vi "Measurement UI.vi"() -> ()   [LabVIEW 2021, in "Sweep_Channel Ganging.lvlib"]
uses:
  Sweep_Channel Ganging.lvlib
panel:
  in  "MeasGraphs":enum32{"I-V Sweep", "Hidden Controls"}(tab)
  out "LoadGraph":T1(graph)
  out "SourceGraph":T2(graph)
  in  "Load measure trigger":string
  in  "Load source trigger":string
  out "Ganged source currents":dbl[](array[numeric])
  out "Ganged source voltages":dbl[](array[numeric])
  out "Ganged load currents":dbl[](array[numeric])
  out "Ganged load voltages":dbl[](array[numeric])
  in  "Load slave resource names":string[](array[string])
  in  "Load master resource name":string
  in  "Source slave resource names":string[](array[string])
  in  "Source master resource name":string
  out "Load sweep points":i32
  out "Source sweep points":i32
  in  "MeasConfigurations":enum32{"Source Config", "Load Config"}(tab)
  in  "Source ON/OFF":bool=TRUE
  in  "Source source delay":dbl=0.005 caption="SOURCE DELAY" format="%.3ps"
  in  "PPSSlaveResourceNames":refnum<k15>[](array[refnum]) caption="SLAVE RESOURCE NAMES"
  in  "PPSMasterResourceName":refnum<k15> caption="MASTER RESOURCE NAME"
  in  "Source stop level":dbl=20.0 caption="STOP LEVEL" format="%#_6pV"
  in  "Source transient response":i32(ring)=1038 caption="TRANSIENT RESPONSE" items=["Slow"=1041, "Normal"=1038, "Fast"=1039]
  in  "Source sense":i32(ring)=1009 caption="SENSE" items=["Local"=1008, "Remote"=1009]
  in  "Source voltage/current level range":dbl=20.0 caption="VOLTAGE LEVEL RANGE" format="%#_6pV"
  in  "Source start level":dbl=6.0 caption="START LEVEL" format="%#_6pV"
  in  "Source current/voltage limit high":dbl=25.0 caption="CURRENT LIMIT/LIMIT HIGH" format="%#_6pA"
  in  "Source current/voltage limit range":dbl=25.0 caption="CURRENT LIMIT RANGE" format="%#_6pA"
  in  "Source limit symmetry":enum32{"Symmetric", "Asymmetric"}(ring)=enum."Asymmetric" caption="LIMIT SYMMETRY"
  in  "Source current/voltage limit low":dbl=-0.6 caption="CURRENT LIMIT LOW" format="%#_6pA"
  in  "Source system configuration":enum32{"Series", "Parallel"}(ring)=enum."Parallel" caption="SYSTEM CONFIG"
  in  "Source compliance":string="Compliance"
  in  "Source sourceadapt":string="SourceAdapt"
  in  "Source sweep points/points per decade":i32=4 caption="PTS/PTS PER DECADE"
  in  "Source output function":i32(ring)=1006 caption="OUTPUT FUNCTION" items=["DC Voltage"=1006, "DC Current"=1007]
  in  "Source timing":string="Timings"
  in  "Source aperture time":dbl=0.01666 caption="APERTURE TIME" format="%.3ps"
  in  "Source sweep scale":string(combo)="Linear" caption="SCALE"
  in  "Load Source Trigger":tag caption="SOURCE TRIGGER"
  in  "Load aperture time":dbl=0.01666 caption="APERTURE TIME" format="%.3ps"
  in  "Load Measure Trigger":tag caption="MEASURE TRIGGER"
  in  "Load trigger config":string="Trigger"
  in  "Load timing":string="Timings"
  in  "Load output function":i32(ring)=1007 caption="OUTPUT FUNCTION" items=["DC Voltage"=1006, "DC Current"=1007]
  in  "Load sweep points/points per decade":i32=10 caption="PTS/PTS PER DECADE"
  in  "Load stop level":dbl=50.0 caption="STOP LEVEL" format="%#_6pA"
  in  "Load sourceadapt":string="SourceAdapt"
  in  "Load compliance":string="Compliance"
  in  "Load system configuration":enum32{"Series", "Parallel"}(ring)=enum."Parallel" caption="SYSTEM CONFIG"
  in  "Load current/voltage limit low":dbl caption="VOLTAGE  LIMIT LOW" format="%#_6pV"
  in  "Load limit symmetry":enum32{"Symmetric", "Asymmetric"}(ring) caption="LIMIT SYMMETRY"
  in  "Load current/voltage limit range":dbl=6.0 caption="VOLTAGE LIMIT RANGE" format="%#_6pV"
  in  "Load current/voltage limit high":dbl=inf caption="VOLTAGE LIMIT/LIMIT HIGH" format="%#_6p"
  in  "Load start level":dbl=2.0 caption="START LEVEL" format="%#_6pA"
  in  "Load voltage/current level range":dbl=80.0 caption="CURRENT LEVEL RANGE" format="%#_6pA"
  in  "Load sense":i32(ring)=1009 caption="SENSE" items=["Local"=1008, "Remote"=1009]
  in  "Load transient response":i32(ring)=1038 caption="TRANSIENT RESPONSE" items=["Slow"=1041, "Normal"=1038, "Fast"=1039]
  in  "LoadSlaveResourceNames":refnum<k15>[](array[refnum]) caption="SLAVE RESOURCE NAMES"
  in  "LoadMasterResourceName":refnum<k15> caption="MASTER RESOURCE NAME"
  in  "Load source delay":dbl=0.005 caption="SOURCE DELAY" format="%.3ps"
  in  "Load sweep scale":string(combo)="Linear" caption="SCALE"
  in  "Load ON/OFF":bool=TRUE
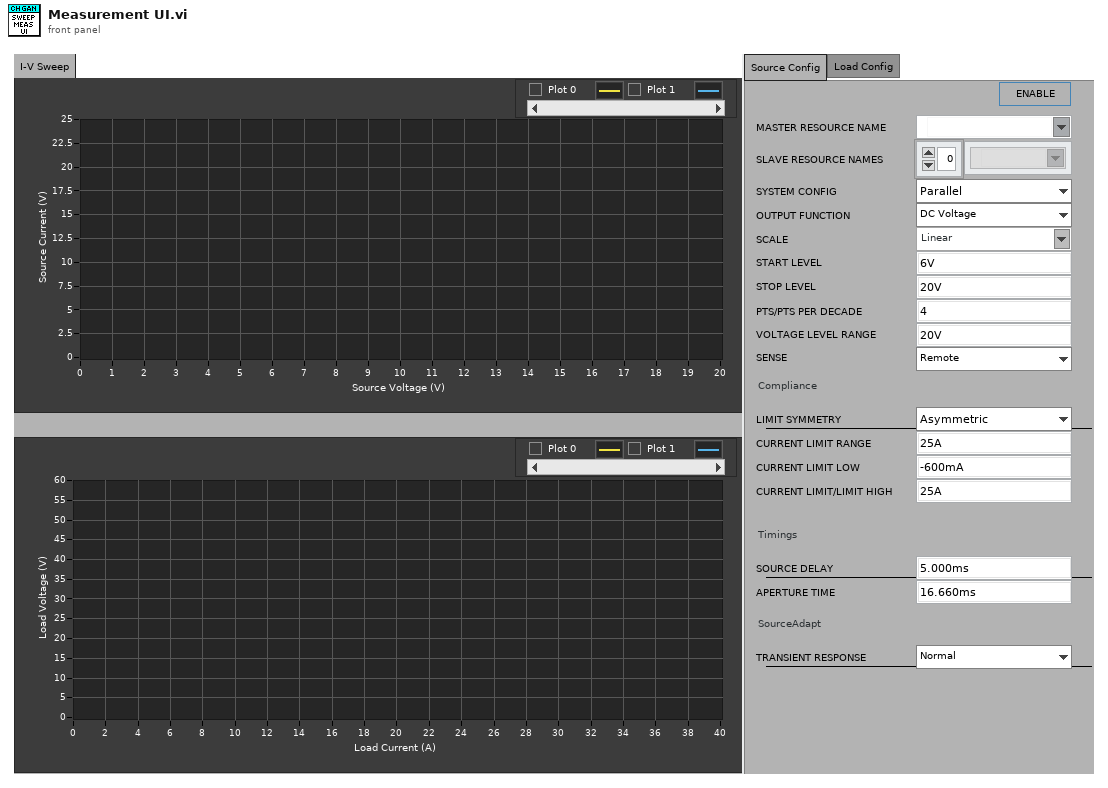
[diagram p1: front panel]
types:
  T1 = cluster{"Ganged load voltages":dbl[], "Ganged load currents":dbl[]}[]
  T2 = cluster{"Ganged source currents":dbl[], "Ganged source voltages":dbl[]}[]
  T3 = cluster{"Ganged source currents":dbl[], "Ganged source voltages":dbl[]}
  T4 = cluster{"Ganged load voltages":dbl[], "Ganged load currents":dbl[]}
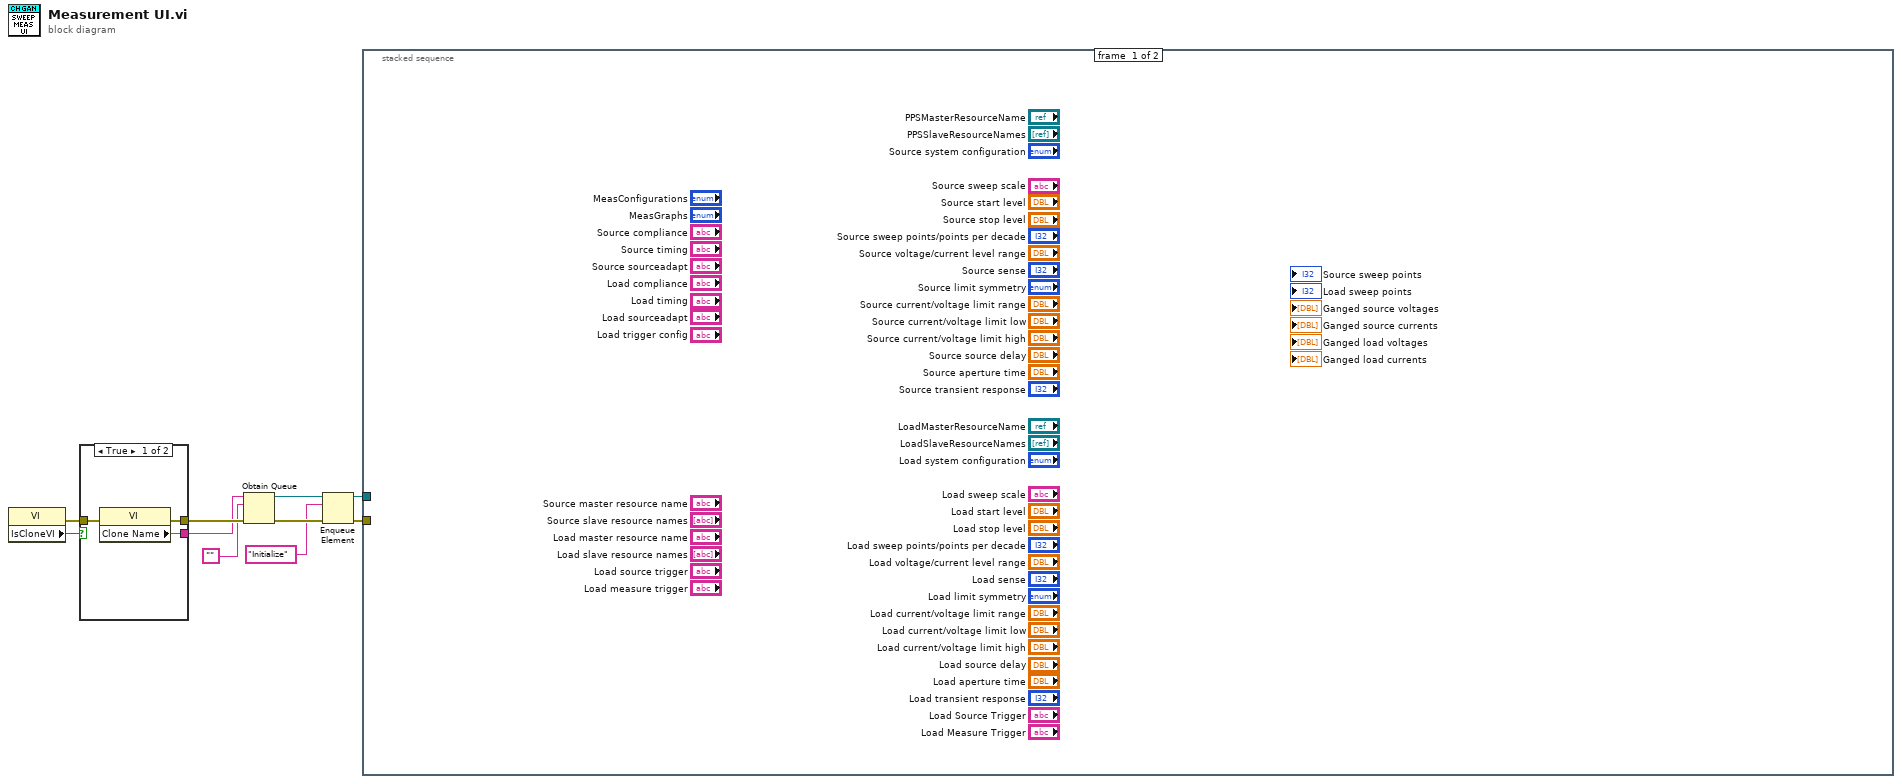
[diagram p0: block diagram]
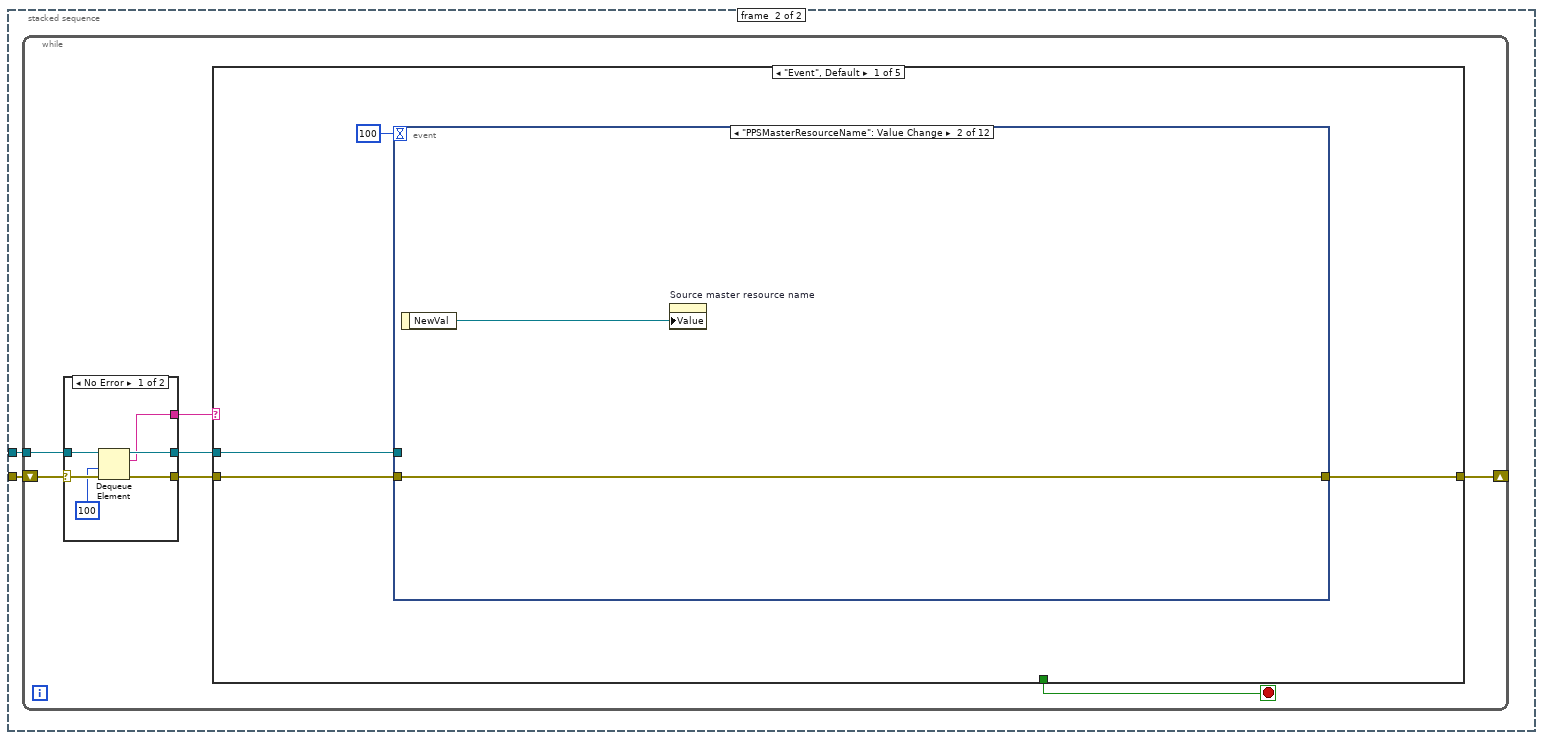
[diagram p2: hidden frame]
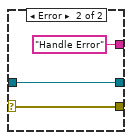
[diagram p3: hidden frame]
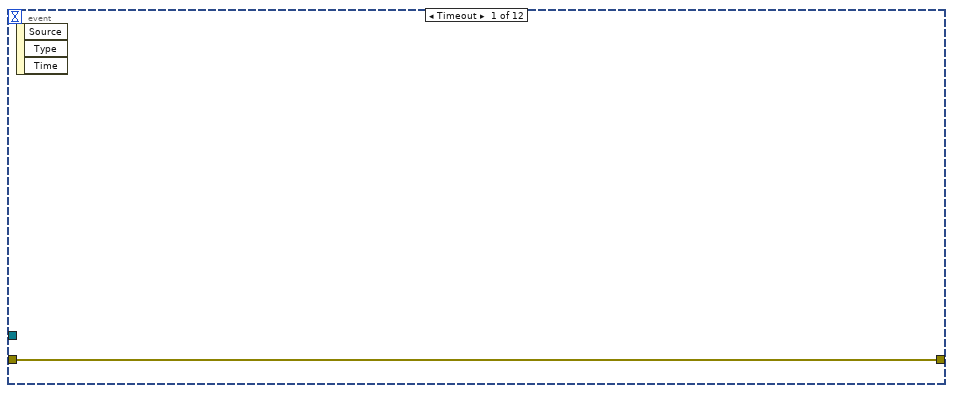
[diagram p4: hidden frame]
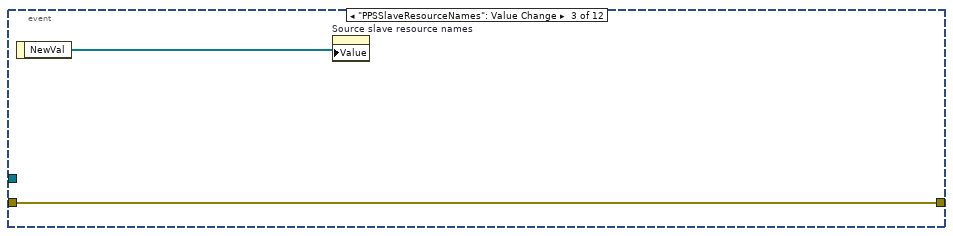
[diagram p5: hidden frame]
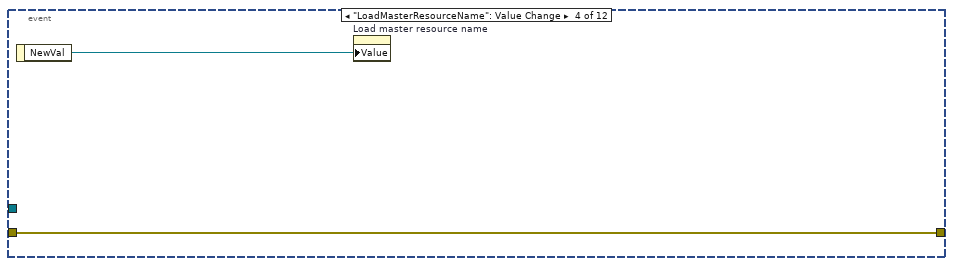
[diagram p6: hidden frame]
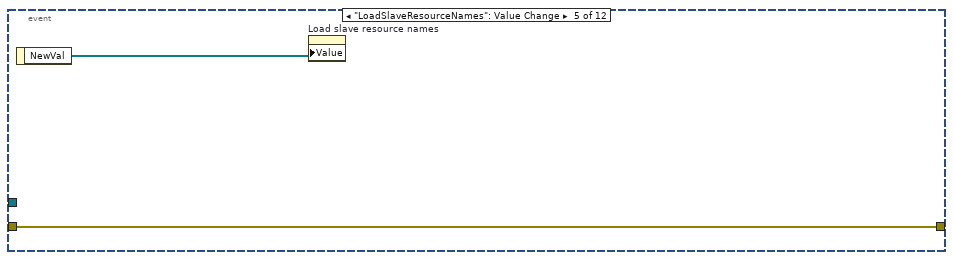
[diagram p7: hidden frame]
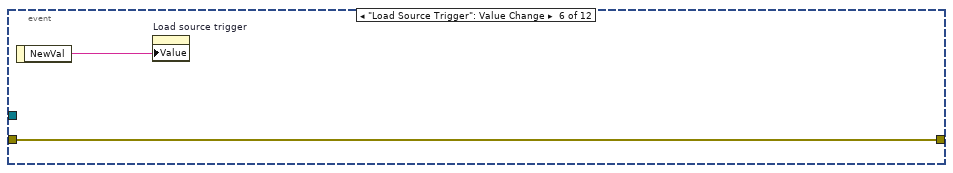
[diagram p8: hidden frame]
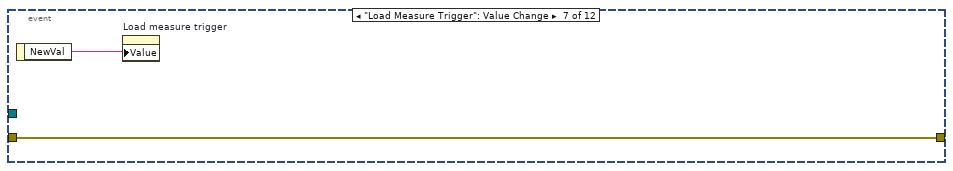
[diagram p9: hidden frame]
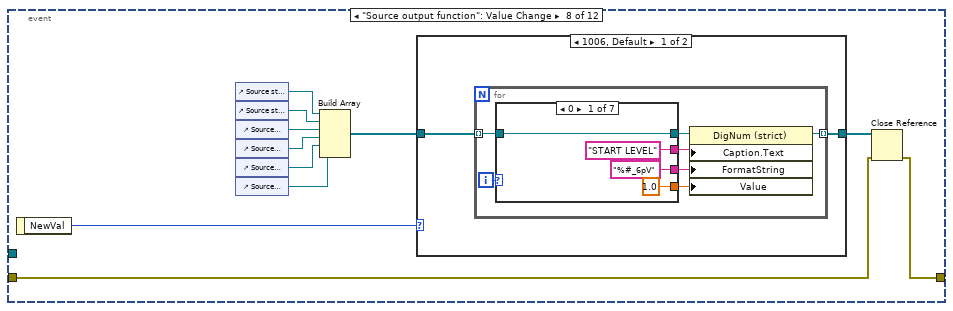
[diagram p10: hidden frame]
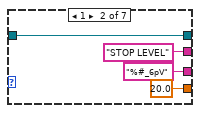
[diagram p11: hidden frame]
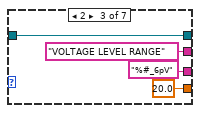
[diagram p12: hidden frame]
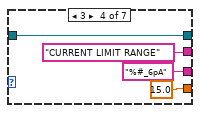
[diagram p13: hidden frame]
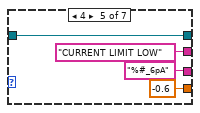
[diagram p14: hidden frame]
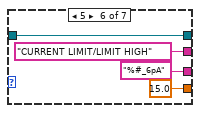
[diagram p15: hidden frame]
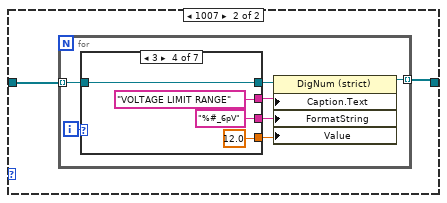
[diagram p17: hidden frame]
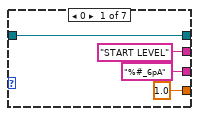
[diagram p18: hidden frame]
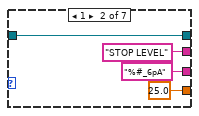
[diagram p19: hidden frame]
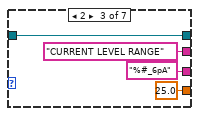
[diagram p20: hidden frame]
diagram:
  n1 = property class="VI"() -> (error out=w1:errorcluster, "IsCloneVI"=w2:bool)  [unwired: 2 in, 1 out]
  n2 = case shown="True" w2 {
    tunnel: [w13 w16] -> w10
    tunnel: [w12 w15] -> w9
    tunnel: w1 -> [w11 w14]
    frame True {
      n3 = property class="VI"(error in=w11) -> (error out=w13:errorcluster, "Clone Name"=w12:string)  [unwired: 1 in, 1 out]
    }
    frame False {
      n4 = property class="VI"(error in=w14) -> (error out=w16:errorcluster, "Name"=w15:string)  [unwired: 1 in, 1 out]
    }
  }
  n5 = Obtain Queue(name (unnamed)=w9, element data type="", error in (no error)=w10) -> (queue out=w6:refnum<queue>, error out=w8:errorcluster)  [unwired: 2 in, 1 out]
  n6 = Enqueue Element(queue=w6, element="Initialize", error in (no error)=w8) -> (queue out=w5:refnum<queue>, error out=w7:errorcluster)  [unwired: 1 in, 1 out]
  n7 = stacked-sequence {
    tunnel: w7 -> [_ w18]
    tunnel: w5 -> [_ w17]
    frame #0 {
    }
    frame #1 {
      n8 = while {
        shift-right: [w20] -> _
        shift-left: w18 -> [w25]
        tunnel: w17 -> [w23]
        stop <- w19 stop-if-true
        n9 = case shown="No Error" w25 {
          selector: w25 -> [w31 w34]
          tunnel: [w30 w34] -> w24
          tunnel: w23 -> [w29 w33]
          tunnel: [w28 w33] -> w22
          tunnel: [w27 "Handle Error"] -> w21
          frame No Error {
            n10 = Dequeue Element(queue=w29, timeout in ms (-1)=100, error in (no error)=w31) -> (queue out=w28:refnum<queue>, element=w27:string, error out=w30:errorcluster)  [unwired: 1 out]
          }
          frame Error {
          }
        }
        n11 = case shown="\"Event\", Default" w21 {
          tunnel: w24 -> [w37 w222 w247 w292 w293]
          tunnel: w22 -> [w35 _ _ w290 _]
          tunnel: [w38 w222 w247 w287 w293] -> w20
          tunnel: [_ _ _ TRUE _] -> w19
          frame "Event", Default {
            n12 = event shown="[1] \"PPSMasterResourceName\": Value Change" {
              selector: _ -> [_ _ _ _ _ _ _ _ _ _ _ _]
              dyn-events: _ -> [_ _ _ _ _ _ _ _ _ _ _ _]
              timeout: 100 -> [_ _ _ _ _ _ _ _ _ _ _ _]
              tunnel: [w39 w41 w43 w44 w46 w48 w50 w52 w129 w207 w212 w219] -> w38
              tunnel: w37 -> [w39 w41 w43 w44 w46 w48 w50 w53 w130 w207 w212 w220]
              tunnel: w35 -> [_ _ _ _ _ _ _ _ _ _ _ w218]
              event Timeout {
                n13 = event-data() -> ()  [unwired: 1 in, 3 out]
              }
              event "PPSMasterResourceName": Value Change {
                n14 = event-data() -> ("NewVal"=w40:refnum<k15>)  [unwired: 1 in]
                n15 = property on="Source master resource name" class="Str"("Value"=w40) -> ()  [unwired: 2 in, 2 out]
              }
              event "PPSSlaveResourceNames": Value Change {
                n16 = event-data() -> ("NewVal"=w42:refnum<k15>[])  [unwired: 1 in]
                n17 = property on="Source slave resource names" class="Arr (strict)"("Value"=w42) -> ()  [unwired: 2 in, 2 out]
              }
              event "LoadMasterResourceName": Value Change {
                n18 = event-data() -> ("NewVal"=w45:refnum<k15>)  [unwired: 1 in]
                n19 = property on="Load master resource name" class="Str"("Value"=w45) -> ()  [unwired: 2 in, 2 out]
              }
              event "LoadSlaveResourceNames": Value Change {
                n20 = event-data() -> ("NewVal"=w47:refnum<k15>[])  [unwired: 1 in]
                n21 = property on="Load slave resource names" class="Arr (strict)"("Value"=w47) -> ()  [unwired: 2 in, 2 out]
              }
              event "Load Source Trigger": Value Change {
                n22 = event-data() -> ("NewVal"=w49:tag)  [unwired: 1 in]
                n23 = property on="Load source trigger" class="Str"("Value"=w49) -> ()  [unwired: 2 in, 2 out]
              }
              event "Load Measure Trigger": Value Change {
                n24 = event-data() -> ("NewVal"=w51:tag)  [unwired: 1 in]
                n25 = property on="Load measure trigger" class="Str"("Value"=w51) -> ()  [unwired: 2 in, 2 out]
              }
              event "Source output function": Value Change {
                n26 = event-data() -> ("NewVal"=w62:i32)  [unwired: 1 in]
                n27 = control-ref of="Source start level"() -> (w61:refnum<vi>)
                n28 = control-ref of="Source stop level"() -> (w60:refnum<vi>)
                n29 = control-ref of="Source voltage/current level range"() -> (w59:refnum<vi>)
                n30 = control-ref of="Source current/voltage limit range"() -> (w58:refnum<vi>)
                n31 = control-ref of="Source current/voltage limit low"() -> (w57:refnum<vi>)
                n32 = control-ref of="Source current/voltage limit high"() -> (w56:refnum<vi>)
                n33 = Build Array(w61, w60, w59, w58, w57, w56) -> (w55:refnum<vi>[])
                n34 = case shown="1006, Default" w62 {
                  tunnel: w55 -> [w64 w97]
                  tunnel: [w63 w96] -> w54
                  frame 1006, Default {
                    n35 = for {
                      tunnel: w64 -> [w69] mode=indexing
                      tunnel: [w65] -> w63 mode=indexing
                      i -> [w71]
                      n36 = case shown="0" w71 {
                        tunnel: [w75 w79 w83 w87 w90 w94 _] -> w70
                        tunnel: w69 -> [w75 w79 w83 w87 w90 w94 _]
                        tunnel: ["START LEVEL" ("Caption.Text") "STOP LEVEL" ("Caption.Text") "VOLTAGE LEVEL RANGE" ("Caption.Text") "CURRENT LIMIT RANGE" ("Caption.Text") "CURRENT LIMIT LOW" ("Caption.Text") "CURRENT LIMIT/LIMIT HIGH" ("Caption.Text") _] -> w68
                        tunnel: ["%#_6pV" ("Format String") "%#_6pV" ("Format String") "%#_6pV" ("Format String") "%#_6pA" ("Format String") "%#_6pA" ("Format String") "%#_6pA" ("Format String") _] -> w67
                        tunnel: [1.0 ("Value") 20.0 ("Value") 20.0 ("Value") 15.0 ("Value") -0.6 ("Value") 15.0 ("Value") _] -> w66
                        frame 0 {
                        }
                        frame 1 {
                        }
                        frame 2 {
                        }
                        frame 3 {
                        }
                        frame 4 {
                        }
                        frame 5 {
                        }
                        frame Default {
                        }
                      }
                      n37 = property class="DigNum (strict)"(reference=w70, "Caption.Text"=w68, "FormatString"=w67, "Value"=w66) -> (reference out=w65:refnum<vi>)  [unwired: 1 in, 1 out]
                    }
                  }
                  frame 1007 {
                    n38 = for {
                      tunnel: w97 -> [w102] mode=indexing
                      tunnel: [w98] -> w96 mode=indexing
                      i -> [w104]
                      n39 = case shown="3" w104 {
                        tunnel: [w108 w112 w116 w120 w123 w127 _] -> w103
                        tunnel: w102 -> [w108 w112 w116 w120 w123 w127 _]
                        tunnel: ["START LEVEL" ("Caption.Text") "STOP LEVEL" ("Caption.Text") "CURRENT LEVEL RANGE" ("Caption.Text") "VOLTAGE LIMIT RANGE" ("Caption.Text") "VOLTAGE  LIMIT LOW" ("Caption.Text") "VOLTAGE LIMIT/LIMIT HIGH" ("Caption.Text") _] -> w101
                        tunnel: ["%#_6pA" ("Format String") "%#_6pA" ("Format String") "%#_6pA" ("Format String") "%#_6pV" ("Format String") "%#_6pV" ("Format String") "%#_6pV" ("Format String") _] -> w100
                        tunnel: [1.0 ("Value") 25.0 ("Value") 25.0 ("Value") 12.0 ("Value") -0.6 ("Value") 12.0 ("Value") _] -> w99
                        frame 0 {
                        }
                        frame 1 {
                        }
                        frame 2 {
                        }
                        frame 3 {
                        }
                        frame 4 {
                        }
                        frame 5 {
                        }
                        frame Default {
                        }
                      }
                      n40 = property class="DigNum (strict)"(reference=w103, "Caption.Text"=w101, "FormatString"=w100, "Value"=w99) -> (reference out=w98:refnum<vi>)  [unwired: 1 in, 1 out]
                    }
                  }
                }
                n41 = Close Reference(reference=w54, error in (no error)=w53) -> (error out=w52:errorcluster)
              }
              event "Load output function": Value Change {
                n42 = event-data() -> ("NewVal"=w139:i32)  [unwired: 1 in]
                n43 = control-ref of="Load start level"() -> (w138:refnum<vi>)
                n44 = control-ref of="Load stop level"() -> (w137:refnum<vi>)
                n45 = control-ref of="Load voltage/current level range"() -> (w135:refnum<vi>)
                n46 = control-ref of="Load current/voltage limit range"() -> (w134:refnum<vi>)
                n47 = control-ref of="Load current/voltage limit low"() -> (w133:refnum<vi>)
                n48 = control-ref of="Load current/voltage limit high"() -> (w132:refnum<vi>)
                n49 = Build Array(w138, w137, w135, w134, w133, w132) -> (w136:refnum<vi>[])
                n50 = case shown="1006" w139 {
                  tunnel: w136 -> [w141 w174]
                  tunnel: [w140 w173] -> w131
                  frame 1006 {
                    n51 = for {
                      tunnel: w141 -> [w146] mode=indexing
                      tunnel: [w142] -> w140 mode=indexing
                      i -> [w148]
                      n52 = case shown="0" w148 {
                        tunnel: [w152 w156 w160 w164 w167 w171 _] -> w147
                        tunnel: w146 -> [w152 w156 w160 w164 w167 w171 _]
                        tunnel: ["START LEVEL" ("Caption.Text") "STOP LEVEL" ("Caption.Text") "VOLTAGE LEVEL RANGE" ("Caption.Text") "CURRENT LIMIT RANGE" ("Caption.Text") "CURRENT LIMIT LOW" ("Caption.Text") "CURRENT LIMIT/LIMIT HIGH" ("Caption.Text") _] -> w145
                        tunnel: ["%#_6pV" ("Format String") "%#_6pV" ("Format String") "%#_6pV" ("Format String") "%#_6pA" ("Format String") "%#_6pA" ("Format String") "%#_6pA" ("Format String") _] -> w144
                        tunnel: [1.0 ("Value") 60.0 ("Value") 60.0 ("Value") 4.0 ("Value") 0.0 ("Value") 4.0 ("Value") _] -> w143
                        frame 0 {
                        }
                        frame 1 {
                        }
                        frame 2 {
                        }
                        frame 3 {
                        }
                        frame 4 {
                        }
                        frame 5 {
                        }
                        frame Default {
                        }
                      }
                      n53 = property class="DigNum (strict)"(reference=w147, "Caption.Text"=w145, "FormatString"=w144, "Value"=w143) -> (reference out=w142:refnum<vi>)  [unwired: 1 in, 1 out]
                    }
                  }
                  frame 1007, Default {
                    n54 = for {
                      tunnel: w174 -> [w179] mode=indexing
                      tunnel: [w175] -> w173 mode=indexing
                      i -> [w181]
                      n55 = case shown="0" w181 {
                        tunnel: [w185 w189 w193 w197 w200 w205 _] -> w180
                        tunnel: w179 -> [w185 w189 w193 w197 w200 w205 _]
                        tunnel: ["START LEVEL" ("Caption.Text") "STOP LEVEL" ("Caption.Text") "CURRENT LEVEL RANGE" ("Caption.Text") "VOLTAGE LIMIT RANGE" ("Caption.Text") "VOLTAGE  LIMIT LOW" ("Caption.Text") "VOLTAGE LIMIT/LIMIT HIGH" ("Caption.Text") _] -> w178
                        tunnel: ["%#_6pA" ("Format String") "%#_6pA" ("Format String") "%#_6pA" ("Format String") "%#_6pV" ("Format String") "%#_6pV" ("Format String") "%#_6p" ("Format String") _] -> w177
                        tunnel: [1.0 ("Value") 40.0 ("Value") 40.0 ("Value") 6.0 ("Value") 0.0 ("Value") w203 _] -> w176
                        frame 0 {
                        }
                        frame 1 {
                        }
                        frame 2 {
                        }
                        frame 3 {
                        }
                        frame 4 {
                        }
                        frame 5 {
                          n56 = Reciprocal(x=0.0) -> (1/x=w203:dbl)
                        }
                        frame Default {
                        }
                      }
                      n57 = property class="DigNum (strict)"(reference=w180, "Caption.Text"=w178, "FormatString"=w177, "Value"=w176) -> (reference out=w175:refnum<vi>)  [unwired: 1 in, 1 out]
                    }
                  }
                }
                n58 = Close Reference(reference=w131, error in (no error)=w130) -> (error out=w129:errorcluster)
              }
              event "Source sweep scale": Value Change {
                n59 = event-data() -> ("NewVal"=w209:string)  [unwired: 1 in]
                n60 = case shown="\"Logarithmic\"" w209 {
                  tunnel: [u8 0 ("X Scale.Mapping Mode") u8 1 ("X Scale.Mapping Mode")] -> w208
                  frame "Linear", Default {
                  }
                  frame "Logarithmic" {
                  }
                }
                n61 = property on="SourceGraph" class="XYGraph (strict)"("XScale.Mapping Mode"=w208) -> ()  [unwired: 2 in, 2 out]
              }
              event "Load sweep scale": Value Change {
                n62 = event-data() -> ("NewVal"=w214:string)  [unwired: 1 in]
                n63 = case shown="\"Logarithmic\"" w214 {
                  tunnel: [u8 0 ("X Scale.Mapping Mode") u8 1 ("X Scale.Mapping Mode")] -> w213
                  frame "Linear", Default {
                  }
                  frame "Logarithmic" {
                  }
                }
                n64 = property on="LoadGraph" class="XYGraph (strict)"("XScale.Mapping Mode"=w213) -> ()  [unwired: 2 in, 2 out]
              }
              event Panel Close? {
                n65 = event-data() -> ()  [unwired: 1 in, 4 out]
                n66 = Enqueue Element(queue=w218, element="Exit", error in (no error)=w220) -> (error out=w219:errorcluster)  [unwired: 1 in, 2 out]
                n67 = event-data("Discard?"=TRUE) -> ()  [unwired: 1 in, 1 out]
              }
            }
          }
          frame "Initialize" {
          }
          frame "Post UI Update" {
            # "Change the X-Scale and Y-Scale label according to the output function given."
            # "This case will be triggered, after framework updates the User interface with result values."
            n68 = local read "Ganged source voltages"() -> (w242:dbl[])
            n69 = local read "Ganged source currents"() -> (w240:dbl[])
            n70 = local read "Ganged load voltages"() -> (w236:dbl[])
            n71 = local read "Ganged load currents"() -> (w237:dbl[])
            n72 = case shown="1006, Default" "Source output function" {
              tunnel: w242 -> [w265 w269]
              tunnel: [w265 w268] -> w241
              tunnel: w240 -> [w264 w268]
              tunnel: [w264 w269] -> w239
              tunnel: ["Source Voltage (V)" ("X Scale.Name Label.Text") "Source Current (A)" ("X Scale.Name Label.Text")] -> w234
              tunnel: ["Source Current (A)" ("X Scale.Name Label.Text") "Source Voltage (V)" ("X Scale.Name Label.Text")] -> w233
              frame 1006, Default {
              }
              frame 1007 {
              }
            }
            n73 = case shown="1007, Default" "Load output function" {
              tunnel: w237 -> [w257 w259]
              tunnel: [w257 w258] -> w238
              tunnel: w236 -> [w256 w258]
              tunnel: [w256 w259] -> w235
              tunnel: ["Load Current (A)" ("X Scale.Name Label.Text") "Load Voltage (V)" ("X Scale.Name Label.Text")] -> w232
              tunnel: ["Load Voltage (V)" ("X Scale.Name Label.Text") "Load Current (A)" ("X Scale.Name Label.Text")] -> w231
              frame 1007, Default {
              }
              frame 1006 {
              }
            }
            n74 = property on="LoadGraph" class="XYGraph (strict)"("XScale.NameLbl.Text"=w232, "YScale.NameLbl.Text"=w231) -> ()  [unwired: 2 in, 2 out]
            n75 = property on="SourceGraph" class="XYGraph (strict)"("XScale.NameLbl.Text"=w234, "YScale.NameLbl.Text"=w233) -> ()  [unwired: 2 in, 2 out]
            n76 = local read "Source sweep points"() -> (w226:i32)
            n77 = local read "Load sweep points"() -> (w224:i32)
            n78 = Build Array("Source ON/OFF", "Load ON/OFF") -> (w227:bool[])
            n79 = Boolean Array To Number(Boolean array=w227) -> (number=w230:u32)
            n80 = case shown="3, Default" w230 {
              tunnel: w226 -> [w249 _ w253]
              tunnel: [1 ("Source sweep points") 1 ("Source sweep points") w253] -> w225
              tunnel: w224 -> [_ w250 w252]
              tunnel: [w249 w250 w252] -> w223
              frame 1 {
              }
              frame 2 {
              }
              frame 3, Default {
              }
            }
            n81 = for {
              N: w225 -> [_]
              tunnel: [w285] -> w245 mode=indexing
              shift-right: [w284] -> _
              shift-left: w241 -> [w281]
              shift-right: [w279] -> _
              shift-left: w239 -> [w280]
              tunnel: w223 -> [w274]
              shift-right: [w272] -> _
              shift-left: w238 -> [w276]
              shift-right: [w271] -> _
              shift-left: w235 -> [w275]
              tunnel: [w270] -> w246 mode=indexing
              w273 = 0 ("index")
              n82 = Delete From Array(array=w281, length=w274, index=w273) -> (deleted portion=w283:dbl[], array with subset deleted=w284:dbl[])
              n83 = Delete From Array(array=w280, length=w274, index=w273) -> (deleted portion=w282:dbl[], array with subset deleted=w279:dbl[])
              n84 = Delete From Array(array=w276, length=w274, index=w273) -> (deleted portion=w277:dbl[], array with subset deleted=w272:dbl[])
              n85 = Delete From Array(array=w275, length=w274, index=w273) -> (deleted portion=w278:dbl[], array with subset deleted=w271:dbl[])
              n86 = Bundle("Ganged source currents"=w283, "Ganged source voltages"=w282) -> (w285:T3)  [unwired: 1 in]
              n87 = Bundle("Ganged load voltages"=w277, "Ganged load currents"=w278) -> (w270:T4)  [unwired: 1 in]
            }
            "LoadGraph" <- w246
            "SourceGraph" <- w245
          }
          frame "Exit" {
            # "This case is triggered to close the User Interface from framework"
            n88 = Flush Queue(queue=w290, error in (no error)=w292) -> (queue out=w289:refnum<queue>, error out=w288:errorcluster)  [unwired: 1 out]
            n89 = Release Queue(queue=w289, force destroy? (F)=TRUE, error in (no error)=w288) -> (error out=w287:errorcluster)  [unwired: 2 out]
          }
          frame "Handle Error" {
          }
        }
      }
    }
  }
